vi "PID_temperature.vi"() -> ()   [LabVIEW 2022 SP3]
uses:
  <vilib>/Analysis/NI_AALBase.lvlib
  <vilib>/addons/control/pid/NI_PID_pid.lvlib
  <vilib>/addons/control/pid/pid.llb/PID Percentage to EGU (DBL).vi
  <vilib>/addons/control/pid/pid.llb/PID (DBL).vi
  <vilib>/Analysis/baseanly.llb/Mean (DBL).vi
panel:
  in  "PID gains":T1={"proportional gain (Kc)"=1.0, "integral time (Ti, min)"=0.01, "derivative time (Td, min)"=0.0} {"derivative time (Td, min)" format="%.3f"; "integral time (Ti, min)" format="%.3f"; "proportional gain (Kc)" format="%.3f"}
  in  "rate (Hz)":dbl
  in  "number of samples":dbl
  out "temperature change (%)":dbl format="%.2f"
  out "temperature-running":cluster{"gewünschte Temperatur (°C)  ":dbl, dbl}(graph)
  in  "reinitialize":bool
  in  "desired temperature (°C)\n(setpoint)":dbl format="%.2f"
  out "voltage output (V)\n(power adapter)":dbl format="%.2f"
  out "measured temperature (°C)\n(process variable)":dbl format="%.2f"
  in  "stop (F)":bool caption="stop PID"
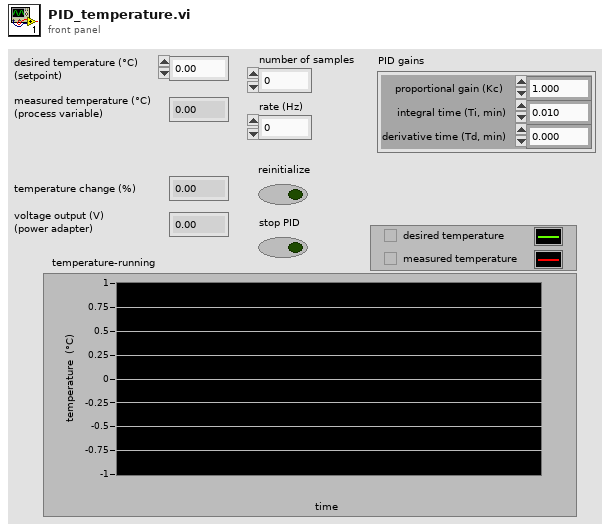
[diagram p1: front panel]
types:
  T1 = cluster{"proportional gain (Kc)":dbl, "integral time (Ti, min)":dbl, "derivative time (Td, min)":dbl}
  T2 = cluster{"desired temperature (°C)\n(setpoint)  ":dbl, "mean":dbl}
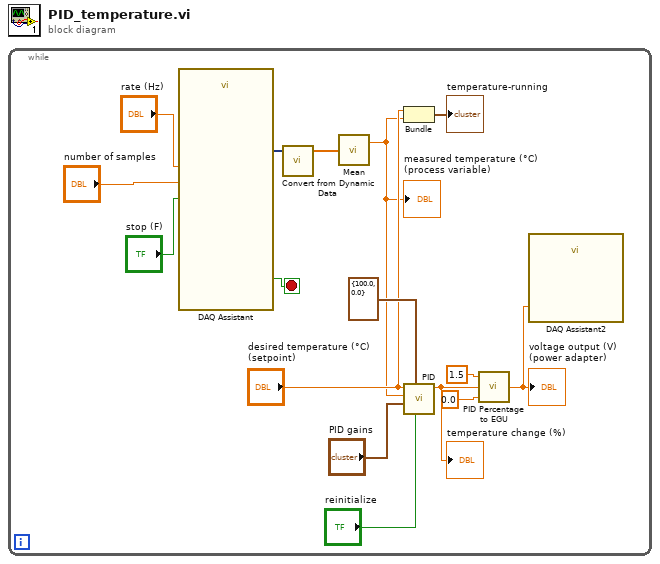
[diagram p0: block diagram]
diagram:
  n1 = while {
    stop <- w1 stop-if-true
    n2 = call "DAQ Assistant"("rate"="rate (Hz)", "number of samples"="number of samples", "stop (F)"="stop (F)") -> ("data"=w5:dynamicdata, "stopped"=w1:bool)  [unwired: 13 in, 2 out]
    n3 = call "Convert from Dynamic Data"("Dynamic Data Type"=w5) -> ("Array"=w16:dbl[])  [unwired: 3 in]
    n4 = call-poly <vilib>:"Mean.vi"("X"=w16) -> ("mean"=w7:dbl)  [unwired: 1 out]
    "measured temperature (°C)\n(process variable)" <- w7
    n5 = Bundle("desired temperature (°C)\n(setpoint)"="desired temperature (°C)\n(setpoint)", "mean"=w7) -> (→"temperature-running":T2)  [unwired: 1 in]
    n6 = call-poly <vilib>:"PID.vi"("reinitialize? (F)"="reinitialize", "output range"=cluster{"output high":dbl, "output low":dbl} {"output high"=100.0, "output low"=0.0}, "PID gains"="PID gains", "process variable"=w7, "setpoint"="desired temperature (°C)\n(setpoint)") -> ("output"=w9:dbl)  [unwired: 5 in, 1 out]
    "temperature change (%)" <- w9
    n7 = call-poly <vilib>:"PID Percentage to EGU.vi"("minimum (EGU)"=0.0 ("Minimum (V)"), "% span"=w9, "maximum (EGU)"=1.5 ("Maximum (V)")) -> ("output (EGU)"=w11:dbl)  [unwired: 1 in]
    "voltage output (V)\n(power adapter)" <- w11
    n8 = call "DAQ Assistant2"("data"=w11) -> ()  [unwired: 17 in, 2 out]
  }
